vi "Shock&Dyanamics Laboratory - DROPBEAR_June2022_Rev3.vi"() -> ()   [LabVIEW 2019] (continued)
                      tunnel: [T42."Disabled and Grayed Out" ("Disabled") T42."Enabled" ("Disabled")] -> _
                      frame False {
                      }
                      frame True {
                      }
                    }
                  }
                  frame "Voltage", Default {
                  }
                }
                n1114 = case shown="\"Strain\"" w1352 {
                  tunnel: [T42."Enabled" ("Disabled") T42."Disabled and Grayed Out" ("Disabled")] -> w1336
                  frame "Strain" {
                    n1115 = property on="SG Pair 17" class="Bool (strict)"() -> ("Value"=w1457:bool)  [unwired: 2 in, 2 out]
                    n1116 = case shown="True" w1457 {
                      tunnel: [T42."Disabled and Grayed Out" ("Disabled") T42."Enabled" ("Disabled")] -> _
                      frame False {
                      }
                      frame True {
                      }
                    }
                  }
                  frame "Voltage", Default {
                  }
                }
                n1117 = case shown="\"Strain\"" w1350 {
                  tunnel: [T42."Enabled" ("Disabled") T42."Disabled and Grayed Out" ("Disabled")] -> w1334
                  frame "Strain" {
                    n1118 = property on="SG Pair 19" class="Bool (strict)"() -> ("Value"=w1447:bool)  [unwired: 2 in, 2 out]
                    n1119 = case shown="True" w1447 {
                      tunnel: [T42."Disabled and Grayed Out" ("Disabled") T42."Enabled" ("Disabled")] -> _
                      frame False {
                      }
                      frame True {
                      }
                    }
                  }
                  frame "Voltage", Default {
                  }
                }
                n1120 = case shown="\"Strain\"" w1384 {
                  tunnel: [T42."Enabled" ("Disabled") T42."Disabled and Grayed Out" ("Disabled")] -> w1381
                  frame "Strain" {
                    n1121 = property on="SG Pair 1" class="Bool (strict)"() -> ("Value"=w1537:bool)  [unwired: 2 in, 2 out]
                    n1122 = case shown="True" w1537 {
                      tunnel: [T42."Disabled and Grayed Out" ("Disabled") T42."Enabled" ("Disabled")] -> _
                      frame False {
                      }
                      frame True {
                      }
                    }
                  }
                  frame "Voltage", Default {
                  }
                }
                n1123 = case shown="\"Strain\"" w1353 {
                  tunnel: [T42."Enabled" ("Disabled") T42."Disabled and Grayed Out" ("Disabled")] -> w1337
                  frame "Strain" {
                    n1124 = property on="SG Pair 16" class="Bool (strict)"() -> ("Value"=w1462:bool)  [unwired: 2 in, 2 out]
                    n1125 = case shown="True" w1462 {
                      tunnel: [T42."Disabled and Grayed Out" ("Disabled") T42."Enabled" ("Disabled")] -> _
                      frame False {
                      }
                      frame True {
                      }
                    }
                  }
                  frame "Voltage", Default {
                  }
                }
                n1126 = case shown="\"Strain\"" w1355 {
                  tunnel: [T42."Enabled" ("Disabled") T42."Disabled and Grayed Out" ("Disabled")] -> w1360
                  frame "Strain" {
                    n1127 = property on="SG Pair 15" class="Bool (strict)"() -> ("Value"=w1467:bool)  [unwired: 2 in, 2 out]
                    n1128 = case shown="True" w1467 {
                      tunnel: [T42."Disabled and Grayed Out" ("Disabled") T42."Enabled" ("Disabled")] -> _
                      frame False {
                      }
                      frame True {
                      }
                    }
                  }
                  frame "Voltage", Default {
                  }
                }
                n1129 = case shown="\"Strain\"" w1386 {
                  tunnel: [T42."Enabled" ("Disabled") T42."Disabled and Grayed Out" ("Disabled")] -> w1385
                  frame "Strain" {
                    n1130 = property on="SG Pair 0" class="Bool (strict)"() -> ("Value"=w1542:bool)  [unwired: 2 in, 2 out]
                    n1131 = case shown="True" w1542 {
                      tunnel: [T42."Disabled and Grayed Out" ("Disabled") T42."Enabled" ("Disabled")] -> _
                      frame False {
                      }
                      frame True {
                      }
                    }
                  }
                  frame "Voltage", Default {
                  }
                }
                n1132 = case shown="\"Strain\"" w1383 {
                  tunnel: [T42."Enabled" ("Disabled") T42."Disabled and Grayed Out" ("Disabled")] -> w1382
                  frame "Strain" {
                    n1133 = property on="SG Pair 2" class="Bool (strict)"() -> ("Value"=w1532:bool)  [unwired: 2 in, 2 out]
                    n1134 = case shown="True" w1532 {
                      tunnel: [T42."Disabled and Grayed Out" ("Disabled") T42."Enabled" ("Disabled")] -> _
                      frame False {
                      }
                      frame True {
                      }
                    }
                  }
                  frame "Voltage", Default {
                  }
                }
                n1135 = case shown="\"Strain\"" w1376 {
                  tunnel: [T42."Enabled" ("Disabled") T42."Disabled and Grayed Out" ("Disabled")] -> w1373
                  frame "Strain" {
                    n1136 = property on="SG Pair 6" class="Bool (strict)"() -> ("Value"=w1512:bool)  [unwired: 2 in, 2 out]
                    n1137 = case shown="True" w1512 {
                      tunnel: [T42."Disabled and Grayed Out" ("Disabled") T42."Enabled" ("Disabled")] -> _
                      frame False {
                      }
                      frame True {
                      }
                    }
                  }
                  frame "Voltage", Default {
                  }
                }
                n1138 = property on="SG Pair 15" class="Bool (strict)"("DisabledEnum"=w1360) -> ()  [unwired: 2 in, 2 out]
                n1139 = property on="SG Pair 27" class="Bool (strict)"("DisabledEnum"=w1326) -> ()  [unwired: 2 in, 2 out]
                n1140 = property on="SG Pair 17" class="Bool (strict)"("DisabledEnum"=w1336) -> ()  [unwired: 2 in, 2 out]
                n1141 = property on="SG Pair 26" class="Bool (strict)"("DisabledEnum"=w1327) -> ()  [unwired: 2 in, 2 out]
                n1142 = property on="SG Pair 28" class="Bool (strict)"("DisabledEnum"=w1322) -> ()  [unwired: 2 in, 2 out]
                n1143 = property on="SG Pair 23" class="Bool (strict)"("DisabledEnum"=w1330) -> ()  [unwired: 2 in, 2 out]
                n1144 = property on="SG Pair 22" class="Bool (strict)"("DisabledEnum"=w1331) -> ()  [unwired: 2 in, 2 out]
                n1145 = property on="SG Pair 25" class="Bool (strict)"("DisabledEnum"=w1328) -> ()  [unwired: 2 in, 2 out]
                n1146 = property on="SG Pair 16" class="Bool (strict)"("DisabledEnum"=w1337) -> ()  [unwired: 2 in, 2 out]
                n1147 = property on="SG Pair 29" class="Bool (strict)"("DisabledEnum"=w1323) -> ()  [unwired: 2 in, 2 out]
                n1148 = property on="SG Pair 24" class="Bool (strict)"("DisabledEnum"=w1329) -> ()  [unwired: 2 in, 2 out]
                n1149 = property on="SG Pair 19" class="Bool (strict)"("DisabledEnum"=w1334) -> ()  [unwired: 2 in, 2 out]
                n1150 = property on="SG Pair 20" class="Bool (strict)"("DisabledEnum"=w1333) -> ()  [unwired: 2 in, 2 out]
                n1151 = property on="SG Pair 30" class="Bool (strict)"("DisabledEnum"=w1324) -> ()  [unwired: 2 in, 2 out]
                n1152 = property on="SG Pair 31" class="Bool (strict)"("DisabledEnum"=w1325) -> ()  [unwired: 2 in, 2 out]
                n1153 = property on="SG Pair 18" class="Bool (strict)"("DisabledEnum"=w1335) -> ()  [unwired: 2 in, 2 out]
                n1154 = property on="SG Pair 21" class="Bool (strict)"("DisabledEnum"=w1332) -> ()  [unwired: 2 in, 2 out]
                n1155 = property on="SG Pair 0" class="Bool (strict)"("DisabledEnum"=w1385) -> ()  [unwired: 2 in, 2 out]
                n1156 = property on="SG Pair 1" class="Bool (strict)"("DisabledEnum"=w1381) -> ()  [unwired: 2 in, 2 out]
                n1157 = property on="SG Pair 2" class="Bool (strict)"("DisabledEnum"=w1382) -> ()  [unwired: 2 in, 2 out]
                n1158 = property on="SG Pair 3" class="Bool (strict)"("DisabledEnum"=w1379) -> ()  [unwired: 2 in, 2 out]
                n1159 = property on="SG Pair 5" class="Bool (strict)"("DisabledEnum"=w1372) -> ()  [unwired: 2 in, 2 out]
                n1160 = property on="SG Pair 4" class="Bool (strict)"("DisabledEnum"=w1371) -> ()  [unwired: 2 in, 2 out]
                n1161 = property on="SG Pair 9" class="Bool (strict)"("DisabledEnum"=w1369) -> ()  [unwired: 2 in, 2 out]
                n1162 = property on="SG Pair 8" class="Bool (strict)"("DisabledEnum"=w1370) -> ()  [unwired: 2 in, 2 out]
                n1163 = property on="SG Pair 6" class="Bool (strict)"("DisabledEnum"=w1373) -> ()  [unwired: 2 in, 2 out]
                n1164 = property on="SG Pair 7" class="Bool (strict)"("DisabledEnum"=w1374) -> ()  [unwired: 2 in, 2 out]
                n1165 = property on="SG Pair 12" class="Bool (strict)"("DisabledEnum"=w1363) -> ()  [unwired: 2 in, 2 out]
                n1166 = property on="SG Pair 10" class="Bool (strict)"("DisabledEnum"=w1368) -> ()  [unwired: 2 in, 2 out]
                n1167 = property on="SG Pair 11" class="Bool (strict)"("DisabledEnum"=w1364) -> ()  [unwired: 2 in, 2 out]
                n1168 = property on="SG Pair 13" class="Bool (strict)"("DisabledEnum"=w1362) -> ()  [unwired: 2 in, 2 out]
                n1169 = property on="SG Pair 14" class="Bool (strict)"("DisabledEnum"=w1361) -> ()  [unwired: 2 in, 2 out]
              }
              event "Load CH Data": Value Change {
                # "Prompt User to Load CH Data File"
                n1170 = event-data() -> ()  [unwired: 1 in, 5 out]
                n1171 = property on="Folder Name to Save Raw Data" class="Str"() -> ("Value"=w1549:string)  [unwired: 2 in, 2 out]
                n1172 = String To Path(string=w1549) -> (path=w1548:path)
                n1173 = File Dialog(4:"XML File" ("pattern label"), 6:"*.xml" ("pattern"), 7:"Load Channel Data File" ("prompt"), 9:"*.xml" ("default name"), 11:w1548) -> (1:w1551:bool, 3:w1550:path)  [unwired: 2 in, 2 out]
                n1174 = case shown="False" w1551 {
                  tunnel: w1550 -> [w2001 _]
                  frame False {
                    n1175 = call "32CHDAQ - Load Channel Data File.vi"("Channel Data File Path"=w2001) -> ("value"=w1820:T43)  [unwired: 13 in, 1 out]
                    n1176 = Unbundle(w1820) -> ("Value"=w1819:T5)  [unwired: 1 out]
                    n1177 = Unbundle(w1820) -> ("Value"=w2000:T44)  [unwired: 1 out]
                    n1178 = Unbundle(w1819) -> ("Value"=w1818:dbl, "Value"=w1817:dbl)  [unwired: 1 out]
                    n1179 = property on="Striker Velocity (m/s)" class="DigNum (strict)"("Value"=w1818) -> ()  [unwired: 2 in, 2 out]
                    n1180 = property on="Sample Rate (Sa/sec)" class="DigNum (strict)"("Value"=w1817) -> ()  [unwired: 2 in, 2 out]
                    n1181 = Unbundle(w2000) -> (w2052:T45, w2051:T46, w1999:T47, w1998:T48, w1997:T49, w1821:T50, w1996:T51, w1995:T4, w1994:T52, w1652:T53, w1653:T54, w1654:T55)
                    n1182 = Unbundle(w1654) -> ("PF Info"=w1835:string, "PF Info"=w1836:string, "PF Info"=w1837:string, "PF Info"=w1838:string, "PF Info"=w1839:string, "PF Info"=w1840:string, "PF Info"=w1841:string, "PF Info"=w1842:string, "PF Info"=w1843:string, "PF Info"=w1844:string, "PF Info"=w1845:string, "PF Info"=w1846:string, "PF Info"=w1847:string, "PF Info"=w1848:string, "PF Info"=w1849:string, "PF Info"=w1850:string, "PF Info 2"=w1602:string, "PF Info 3"=w1601:string, "PF Info 4"=w1600:string, "PF Info 5"=w1599:string, "PF Info 6"=w1598:string, "PF Info 7"=w1597:string, "PF Info 8"=w1596:string, "PF Info 9"=w1595:string, "PF Info 10"=w1594:string, "PF Info 11"=w1593:string, "PF Info 12"=w1592:string, "PF Info 13"=w1591:string, "PF Info 14"=w1590:string, "PF Info 15"=w1589:string, "PF Info 16"=w1588:string, "PF Info 17"=w1603:string)
                    n1183 = call "32CHDAQ - PF Info Str2Num.vi"("PF Info"=w1835) -> ("PF Channel"=w2047:dbl, "PF Card"=w2048:dbl, "PF Chassis"=w2049:dbl)  [unwired: 2 in]
                    n1184 = call "32CHDAQ - PF Info Str2Num.vi"("PF Info"=w1836) -> ("PF Channel"=w2044:dbl, "PF Card"=w2045:dbl, "PF Chassis"=w2046:dbl)  [unwired: 2 in]
                    n1185 = call "32CHDAQ - PF Info Str2Num.vi"("PF Info"=w1837) -> ("PF Channel"=w2004:dbl, "PF Card"=w2003:dbl, "PF Chassis"=w2002:dbl)  [unwired: 2 in]
                    n1186 = call "32CHDAQ - PF Info Str2Num.vi"("PF Info"=w1838) -> ("PF Channel"=w2007:dbl, "PF Card"=w2006:dbl, "PF Chassis"=w2005:dbl)  [unwired: 2 in]
                    n1187 = call "32CHDAQ - PF Info Str2Num.vi"("PF Info"=w1839) -> ("PF Channel"=w2010:dbl, "PF Card"=w2009:dbl, "PF Chassis"=w2008:dbl)  [unwired: 2 in]
                    n1188 = call "32CHDAQ - PF Info Str2Num.vi"("PF Info"=w1841) -> ("PF Channel"=w2016:dbl, "PF Card"=w2015:dbl, "PF Chassis"=w2014:dbl)  [unwired: 2 in]
                    n1189 = call "32CHDAQ - PF Info Str2Num.vi"("PF Info"=w1842) -> ("PF Channel"=w2019:dbl, "PF Card"=w2018:dbl, "PF Chassis"=w2017:dbl)  [unwired: 2 in]
                    n1190 = call "32CHDAQ - PF Info Str2Num.vi"("PF Info"=w1843) -> ("PF Channel"=w2022:dbl, "PF Card"=w2021:dbl, "PF Chassis"=w2020:dbl)  [unwired: 2 in]
                    n1191 = call "32CHDAQ - PF Info Str2Num.vi"("PF Info"=w1844) -> ("PF Channel"=w2025:dbl, "PF Card"=w2024:dbl, "PF Chassis"=w2023:dbl)  [unwired: 2 in]
                    n1192 = call "32CHDAQ - PF Info Str2Num.vi"("PF Info"=w1845) -> ("PF Channel"=w2028:dbl, "PF Card"=w2027:dbl, "PF Chassis"=w2026:dbl)  [unwired: 2 in]
                    n1193 = call "32CHDAQ - PF Info Str2Num.vi"("PF Info"=w1846) -> ("PF Channel"=w2031:dbl, "PF Card"=w2030:dbl, "PF Chassis"=w2029:dbl)  [unwired: 2 in]
                    n1194 = call "32CHDAQ - PF Info Str2Num.vi"("PF Info"=w1847) -> ("PF Channel"=w2034:dbl, "PF Card"=w2033:dbl, "PF Chassis"=w2032:dbl)  [unwired: 2 in]
                    n1195 = call "32CHDAQ - PF Info Str2Num.vi"("PF Info"=w1848) -> ("PF Channel"=w2037:dbl, "PF Card"=w2036:dbl, "PF Chassis"=w2035:dbl)  [unwired: 2 in]
                    n1196 = call "32CHDAQ - PF Info Str2Num.vi"("PF Info"=w1849) -> ("PF Channel"=w2040:dbl, "PF Card"=w2039:dbl, "PF Chassis"=w2038:dbl)  [unwired: 2 in]
                    n1197 = call "32CHDAQ - PF Info Str2Num.vi"("PF Info"=w1850) -> ("PF Channel"=w2041:dbl, "PF Card"=w2042:dbl, "PF Chassis"=w2043:dbl)  [unwired: 2 in]
                    n1198 = call "32CHDAQ - PF Info Str2Num.vi"("PF Info"=w1602) -> ("PF Channel"=w1649:dbl, "PF Card"=w1650:dbl, "PF Chassis"=w1651:dbl)  [unwired: 2 in]
                    n1199 = call "32CHDAQ - PF Info Str2Num.vi"("PF Info"=w1601) -> ("PF Channel"=w1646:dbl, "PF Card"=w1647:dbl, "PF Chassis"=w1648:dbl)  [unwired: 2 in]
                    n1200 = call "32CHDAQ - PF Info Str2Num.vi"("PF Info"=w1600) -> ("PF Channel"=w1643:dbl, "PF Card"=w1644:dbl, "PF Chassis"=w1645:dbl)  [unwired: 2 in]
                    n1201 = call "32CHDAQ - PF Info Str2Num.vi"("PF Info"=w1599) -> ("PF Channel"=w1640:dbl, "PF Card"=w1641:dbl, "PF Chassis"=w1642:dbl)  [unwired: 2 in]
                    n1202 = call "32CHDAQ - PF Info Str2Num.vi"("PF Info"=w1598) -> ("PF Channel"=w1637:dbl, "PF Card"=w1638:dbl, "PF Chassis"=w1639:dbl)  [unwired: 2 in]
                    n1203 = call "32CHDAQ - PF Info Str2Num.vi"("PF Info"=w1596) -> ("PF Channel"=w1631:dbl, "PF Card"=w1632:dbl, "PF Chassis"=w1633:dbl)  [unwired: 2 in]
                    n1204 = call "32CHDAQ - PF Info Str2Num.vi"("PF Info"=w1595) -> ("PF Channel"=w1628:dbl, "PF Card"=w1629:dbl, "PF Chassis"=w1630:dbl)  [unwired: 2 in]
                    n1205 = call "32CHDAQ - PF Info Str2Num.vi"("PF Info"=w1594) -> ("PF Channel"=w1625:dbl, "PF Card"=w1626:dbl, "PF Chassis"=w1627:dbl)  [unwired: 2 in]
                    n1206 = call "32CHDAQ - PF Info Str2Num.vi"("PF Info"=w1593) -> ("PF Channel"=w1622:dbl, "PF Card"=w1623:dbl, "PF Chassis"=w1624:dbl)  [unwired: 2 in]
                    n1207 = call "32CHDAQ - PF Info Str2Num.vi"("PF Info"=w1592) -> ("PF Channel"=w1619:dbl, "PF Card"=w1620:dbl, "PF Chassis"=w1621:dbl)  [unwired: 2 in]
                    n1208 = call "32CHDAQ - PF Info Str2Num.vi"("PF Info"=w1591) -> ("PF Channel"=w1616:dbl, "PF Card"=w1617:dbl, "PF Chassis"=w1618:dbl)  [unwired: 2 in]
                    n1209 = call "32CHDAQ - PF Info Str2Num.vi"("PF Info"=w1590) -> ("PF Channel"=w1613:dbl, "PF Card"=w1614:dbl, "PF Chassis"=w1615:dbl)  [unwired: 2 in]
                    n1210 = call "32CHDAQ - PF Info Str2Num.vi"("PF Info"=w1589) -> ("PF Channel"=w1610:dbl, "PF Card"=w1611:dbl, "PF Chassis"=w1612:dbl)  [unwired: 2 in]
                    n1211 = call "32CHDAQ - PF Info Str2Num.vi"("PF Info"=w1588) -> ("PF Channel"=w1607:dbl, "PF Card"=w1608:dbl, "PF Chassis"=w1609:dbl)  [unwired: 2 in]
                    n1212 = call "32CHDAQ - PF Info Str2Num.vi"("PF Info"=w1603) -> ("PF Channel"=w1604:dbl, "PF Card"=w1605:dbl, "PF Chassis"=w1606:dbl)  [unwired: 2 in]
                    n1213 = call "32CHDAQ - PF Info Str2Num.vi"("PF Info"=w1840) -> ("PF Channel"=w2013:dbl, "PF Card"=w2012:dbl, "PF Chassis"=w2011:dbl)  [unwired: 2 in]
                    n1214 = call "32CHDAQ - PF Info Str2Num.vi"("PF Info"=w1597) -> ("PF Channel"=w1634:dbl, "PF Card"=w1635:dbl, "PF Chassis"=w1636:dbl)  [unwired: 2 in]
                    n1215 = local write "PF Chassis 26"(w1621) -> ()
                    n1216 = local write "PF Channel 26"(w1619) -> ()
                    n1217 = local write "PF Channel 22"(w1631) -> ()
                    n1218 = local write "PF Chassis 21"(w1636) -> ()
                    n1219 = local write "PF Chassis 27"(w1618) -> ()
                    n1220 = local write "PF Chassis 23"(w1630) -> ()
                    n1221 = local write "PF Channel 23"(w1628) -> ()
                    n1222 = local write "PF Chassis 24"(w1627) -> ()
                    n1223 = local write "PF Channel 24"(w1625) -> ()
                    n1224 = local write "PF Channel 19"(w1640) -> ()
                    n1225 = local write "PF Chassis 20"(w1639) -> ()
                    n1226 = local write "PF Channel 20"(w1637) -> ()
                    n1227 = local write "PF Chassis 22"(w1633) -> ()
                    n1228 = local write "PF Channel 21"(w1634) -> ()
                    n1229 = local write "PF Channel 25"(w1622) -> ()
                    n1230 = local write "PF Channel 18"(w1643) -> ()
                    n1231 = local write "PF Chassis 25"(w1624) -> ()
                    n1232 = local write "PF Card 26"(w1620) -> ()
                    n1233 = local write "PF Chassis 19"(w1642) -> ()
                    n1234 = local write "PF Channel 27"(w1616) -> ()
                    n1235 = local write "PF Channel 28"(w1613) -> ()
                    n1236 = local write "PF Chassis 0"(w2049) -> ()
                    n1237 = local write "PF Card 0"(w2048) -> ()
                    n1238 = local write "PF Channel 0"(w2047) -> ()
                    n1239 = local write "PF Chassis 1"(w2046) -> ()
                    n1240 = local write "PF Card 1"(w2045) -> ()
                    n1241 = local write "PF Channel 1"(w2044) -> ()
                    n1242 = local write "PF Chassis 2"(w2002) -> ()
                    n1243 = local write "PF Card 2"(w2003) -> ()
                    n1244 = local write "PF Channel 2"(w2004) -> ()
                    n1245 = local write "PF Chassis 3"(w2005) -> ()
                    n1246 = local write "PF Card 3"(w2006) -> ()
                    n1247 = local write "PF Channel 3"(w2007) -> ()
                    n1248 = local write "PF Chassis 4"(w2008) -> ()
                    n1249 = local write "PF Card 4"(w2009) -> ()
                    n1250 = local write "PF Channel 4"(w2010) -> ()
                    n1251 = local write "PF Chassis 6"(w2014) -> ()
                    n1252 = local write "PF Card 6"(w2015) -> ()
                    n1253 = local write "PF Channel 6"(w2016) -> ()
                    n1254 = local write "PF Chassis 7"(w2017) -> ()
                    n1255 = local write "PF Card 7"(w2018) -> ()
                    n1256 = local write "PF Channel 7"(w2019) -> ()
                    n1257 = local write "PF Chassis 8"(w2020) -> ()
                    n1258 = local write "PF Channel 8"(w2021) -> ()
                    n1259 = local write "PF Card 8"(w2022) -> ()
                    n1260 = local write "PF Chassis 9"(w2023) -> ()
                    n1261 = local write "PF Card 9"(w2024) -> ()
                    n1262 = local write "PF Channel 9"(w2025) -> ()
                    n1263 = local write "PF Chassis 10"(w2026) -> ()
                    n1264 = local write "PF Card 10"(w2027) -> ()
                    n1265 = local write "PF Channel 10"(w2028) -> ()
                    n1266 = local write "PF Chassis 11"(w2029) -> ()
                    n1267 = local write "PF Card 11"(w2030) -> ()
                    n1268 = local write "PF Channel 11"(w2031) -> ()
                    n1269 = local write "PF Chassis 12"(w2032) -> ()
                    n1270 = local write "PF Card 12"(w2033) -> ()
                    n1271 = local write "PF Channel 12"(w2034) -> ()
                    n1272 = local write "PF Chassis 13"(w2035) -> ()
                    n1273 = local write "PF Card 13"(w2036) -> ()
                    n1274 = local write "PF Channel 13"(w2037) -> ()
                    n1275 = local write "PF Chassis 14"(w2038) -> ()
                    n1276 = local write "PF Card 14"(w2039) -> ()
                    n1277 = local write "PF Channel 14"(w2040) -> ()
                    n1278 = local write "PF Chassis 15"(w2043) -> ()
                    n1279 = local write "PF Card 15"(w2042) -> ()
                    n1280 = local write "PF Channel 15"(w2041) -> ()
                    n1281 = local write "PF Channel 17"(w1646) -> ()
                    n1282 = local write "PF Chassis 28"(w1615) -> ()
                    n1283 = local write "PF Chassis 29"(w1612) -> ()
                    n1284 = local write "PF Chassis 16"(w1651) -> ()
                    n1285 = local write "PF Channel 16"(w1649) -> ()
                    n1286 = local write "PF Chassis 18"(w1645) -> ()
                    n1287 = local write "PF Channel 29"(w1610) -> ()
                    n1288 = local write "PF Chassis 30"(w1609) -> ()
                    n1289 = local write "PF Chassis 17"(w1648) -> ()
                    n1290 = local write "PF Card 23"(w1629) -> ()
                    n1291 = local write "PF Channel 30"(w1607) -> ()
                    n1292 = local write "PF Card 21"(w1635) -> ()
                    n1293 = local write "PF Card 24"(w1626) -> ()
                    n1294 = local write "PF Chassis 5"(w2011) -> ()
                    n1295 = local write "PF Card 5"(w2012) -> ()
                    n1296 = local write "PF Channel 5"(w2013) -> ()
                    n1297 = local write "PF Card 22"(w1632) -> ()
                    n1298 = local write "PF Card 16"(w1650) -> ()
                    n1299 = local write "PF Card 20"(w1638) -> ()
                    n1300 = local write "PF Card 27"(w1617) -> ()
                    n1301 = local write "PF Chassis 31"(w1606) -> ()
                    n1302 = local write "PF Card 17"(w1647) -> ()
                    n1303 = local write "PF Card 19"(w1641) -> ()
                    n1304 = local write "PF Card 28"(w1614) -> ()
                    n1305 = local write "PF Card 29"(w1611) -> ()
                    n1306 = local write "PF Card 18"(w1644) -> ()
                    n1307 = local write "PF Card 25"(w1623) -> ()
                    n1308 = local write "PF Card 30"(w1608) -> ()
                    n1309 = local write "PF Channel 31"(w1604) -> ()
                    n1310 = Unbundle(w2052) -> ("Enable Ch 1"=w1834:bool, "Enable Ch 2"=w1833:bool, "Enable Ch 3"=w1832:bool, "Enable Ch 4"=w1831:bool, "Enable Ch 5"=w1830:bool, "Enable Ch 6"=w1829:bool, "Enable Ch 7"=w1828:bool, "Enable Ch 8"=w1827:bool, "Enable Ch 9"=w1826:bool, "Enable Ch 10"=w1825:bool, "Enable Ch 11"=w1824:bool, "Enable Ch 12"=w1823:bool, "Enable Ch 13"=w1822:bool, "Enable Ch 14"=w1816:bool, "Enable Ch 15"=w1815:bool, "Enable Ch 16"=w1814:bool, "Enable Ch 17"=w1813:bool, "Enable Ch 18"=w1812:bool, "Enable Ch 19"=w1811:bool, "Enable Ch 20"=w1810:bool, "Enable Ch 21"=w1799:bool, "Enable Ch 22"=w1800:bool, "Enable Ch 23"=w1801:bool, "Enable Ch 24"=w1802:bool, "Enable Ch 25"=w1803:bool, "Enable Ch 26"=w1804:bool, "Enable Ch 27"=w1805:bool, "Enable Ch 28"=w1806:bool, "Enable Ch 29"=w1807:bool, "Enable Ch 30"=w1808:bool, w1809:bool)  [unwired: 1 out]
                    n1311 = local write "PF Card 31"(w1605) -> ()
                    n1312 = property on="Enable Ch 12" class="Bool (strict)"("Value"=w1823) -> ()  [unwired: 2 in, 2 out]
                    n1313 = property on="Enable Ch 13" class="Bool (strict)"("Value"=w1822) -> ()  [unwired: 2 in, 2 out]
                    n1314 = property on="Enable Ch 15" class="Bool (strict)"("Value"=w1815) -> ()  [unwired: 2 in, 2 out]
                    n1315 = property on="Enable Ch 11" class="Bool (strict)"("Value"=w1824) -> ()  [unwired: 2 in, 2 out]
                    n1316 = property on="Enable Ch 14" class="Bool (strict)"("Value"=w1816) -> ()  [unwired: 2 in, 2 out]
                    n1317 = property on="Enable Ch 10" class="Bool (strict)"("Value"=w1825) -> ()  [unwired: 2 in, 2 out]
                    n1318 = property on="Enable Ch 9" class="Bool (strict)"("Value"=w1826) -> ()  [unwired: 2 in, 2 out]
                    n1319 = property on="Enable Ch 6" class="Bool (strict)"("Value"=w1829) -> ()  [unwired: 2 in, 2 out]
                    n1320 = property on="Enable Ch 4" class="Bool (strict)"("Value"=w1831) -> ()  [unwired: 2 in, 2 out]
                    n1321 = property on="Enable Ch 5" class="Bool (strict)"("Value"=w1830) -> ()  [unwired: 2 in, 2 out]
                    n1322 = property on="Enable Ch 7" class="Bool (strict)"("Value"=w1828) -> ()  [unwired: 2 in, 2 out]
                    n1323 = property on="Enable Ch 8" class="Bool (strict)"("Value"=w1827) -> ()  [unwired: 2 in, 2 out]
                    n1324 = property on="Enable Ch 3" class="Bool (strict)"("Value"=w1832) -> ()  [unwired: 2 in, 2 out]
                    n1325 = property on="Enable Ch 1" class="Bool (strict)"("Value"=w1834) -> ()  [unwired: 2 in, 2 out]
                    n1326 = property on="Enable Ch 2" class="Bool (strict)"("Value"=w1833) -> ()  [unwired: 2 in, 2 out]
                    n1327 = local write "LED Enable Ch 18"(w1812) -> ()
                    n1328 = local write "LED Enable Ch 16"(w1814) -> ()
                    n1329 = local write "LED Enable Ch 12"(w1823) -> ()
                    n1330 = local write "LED Enable Ch 17"(w1813) -> ()
                    n1331 = local write "LED Enable Ch 19"(w1811) -> ()
                    n1332 = local write "LED Enable Ch 9"(w1826) -> ()
                    n1333 = local write "LED Enable Ch 13"(w1822) -> ()
                    n1334 = local write "LED Enable Ch 20"(w1810) -> ()
                    n1335 = local write "LED Enable Ch 10"(w1825) -> ()
                    n1336 = local write "LED Enable Ch 11"(w1824) -> ()
                    n1337 = local write "LED Enable Ch 6"(w1829) -> ()
                    n1338 = local write "LED Enable Ch 7"(w1828) -> ()
                    n1339 = local write "LED Enable Ch 5"(w1830) -> ()
                    n1340 = local write "LED Enable Ch 8"(w1827) -> ()
                    n1341 = local write "LED Enable Ch 4"(w1831) -> ()
                    n1342 = local write "LED Enable Ch 3"(w1832) -> ()
                    n1343 = local write "LED Enable Ch 14"(w1816) -> ()
                    n1344 = local write "LED Enable Ch 15"(w1815) -> ()
                    n1345 = local write "LED Enable Ch 1"(w1834) -> ()
                    n1346 = local write "LED Enable Ch 2"(w1833) -> ()
                    n1347 = local write "LED Enable Ch 22"(w1800) -> ()
                    n1348 = local write "LED Enable Ch 23"(w1801) -> ()
                    n1349 = local write "LED Enable Ch 24"(w1802) -> ()
                    n1350 = local write "LED Enable Ch 21"(w1799) -> ()
                    n1351 = Unbundle(w1653) -> ("PF Condition 0"=w1866:bool, "PF Condition 1"=w1863:bool, "PF Condition 2"=w1861:bool, "PF Condition 3"=w1860:bool, "PF Condition 4"=w1859:bool, "PF Condition 5"=w1854:bool, "PF Condition 6"=w1853:bool, "PF Condition 7"=w1852:bool, "PF Condition 8"=w1851:bool, "PF Condition 9"=w1855:bool, "PF Condition 10"=w1856:bool, "PF Condition 11"=w1857:bool, "PF Condition 12"=w1858:bool, "PF Condition 13"=w1862:bool, "PF Condition 14"=w1864:bool, "PF Condition 15"=w1865:bool, "PF Condition 16"=w1686:bool, "PF Condition 17"=w1685:bool, "PF Condition 18"=w1684:bool, "PF Condition 19"=w1683:bool, "PF Condition 20"=w1682:bool, "PF Condition 21"=w1681:bool, "PF Condition 22"=w1680:bool, "PF Condition 23"=w1679:bool, "PF Condition 24"=w1678:bool, "PF Condition 25"=w1677:bool, "PF Condition 26"=w1676:bool, "PF Condition 27"=w1675:bool, "PF Condition 28"=w1674:bool, "PF Condition 29"=w1673:bool, "PF Condition 30"=w1672:bool, "PF Condition 31"=w1671:bool)
                    n1352 = local write "LED Enable Ch 25"(w1803) -> ()
                    n1353 = local write "LED Enable Ch 26"(w1804) -> ()
                    n1354 = local write "LED Enable Ch 28"(w1806) -> ()
                    n1355 = local write "LED Enable Ch 27"(w1805) -> ()
                    n1356 = local write "LED Enable Ch 29"(w1807) -> ()
                    n1357 = local write "LED Enable Ch 30"(w1808) -> ()
                    n1358 = local write "LED Enable Ch 31"(w1809) -> ()
                    n1359 = local write "PF Condition 0"(w1866) -> ()
                    n1360 = local write "PF Condition 1"(w1863) -> ()
                    n1361 = local write "PF Condition 2"(w1861) -> ()
                    n1362 = local write "PF Condition 3"(w1860) -> ()
                    n1363 = local write "PF Condition 4"(w1859) -> ()
                    n1364 = local write "PF Condition 5"(w1854) -> ()
                    n1365 = local write "PF Condition 6"(w1853) -> ()
                    n1366 = local write "PF Condition 7"(w1852) -> ()
                    n1367 = local write "PF Condition 8"(w1851) -> ()
                    n1368 = local write "PF Condition 9"(w1855) -> ()
                    n1369 = local write "PF Condition 10"(w1856) -> ()
                    n1370 = local write "PF Condition 11"(w1857) -> ()
                    n1371 = local write "PF Condition 12"(w1858) -> ()
                    n1372 = local write "PF Condition 13"(w1862) -> ()
                    n1373 = local write "PF Condition 14"(w1864) -> ()
                    n1374 = local write "PF Condition 15"(w1865) -> ()
                    n1375 = local write "PF Condition 28"(w1674) -> ()
                    n1376 = local write "PF Condition 29"(w1673) -> ()
                    n1377 = local write "PF Condition 23"(w1679) -> ()
                    n1378 = local write "PF Condition 16"(w1686) -> ()
                    n1379 = local write "PF Condition 20"(w1682) -> ()
                    n1380 = local write "PF Condition 21"(w1681) -> ()
                    n1381 = local write "PF Condition 24"(w1678) -> ()
                    n1382 = local write "PF Condition 17"(w1685) -> ()
                    n1383 = local write "PF Condition 18"(w1684) -> ()
                    n1384 = local write "PF Condition 22"(w1680) -> ()
                    n1385 = local write "PF Condition 25"(w1677) -> ()
                    n1386 = local write "PF Condition 26"(w1676) -> ()
                    n1387 = local write "PF Condition 27"(w1675) -> ()
                    n1388 = local write "PF Condition 19"(w1683) -> ()
                    n1389 = local write "PF Condition 30"(w1672) -> ()
                    n1390 = local write "PF Condition 31"(w1671) -> ()
                    n1391 = Unbundle(w2051) -> ("Name (Trigger Channel)"=w2050:string, "Name Ch 1"=w1979:string, "Name Ch 2"=w1980:string, "Name Ch 3"=w1981:string, "Name Ch4"=w1982:string, "Name Ch 5"=w1983:string, "Name Ch 6"=w1984:string, "Name Ch 7"=w1985:string, "Name Ch 8"=w1986:string, "Name Ch 9"=w1987:string, "Name Ch 10"=w1988:string, "Name Ch 11"=w1989:string, "Name Ch 12"=w1990:string, "Name Ch 13"=w1991:string, "Name Ch 14"=w1992:string, "Name Ch 15"=w1993:string, "Name Ch 16"=w1798:string, "Name Ch 17"=w1797:string, "Name Ch 18"=w1796:string, "Name Ch 19"=w1795:string, "Name Ch 20"=w1794:string, "Name Ch 21"=w1793:string, "Name Ch 22"=w1792:string, "Name Ch 23"=w1791:string, "Name Ch 24"=w1790:string, "Name Ch 25"=w1789:string, "Name Ch 26"=w1788:string, "Name Ch4 2"=w1787:string, "Name Ch 4"=w1786:string, "Name Ch 27"=w1785:string, "Name Ch 28"=w1784:string, "Name (Trigger Channel) 2"=w1783:string)
                    n1392 = local write "Name Ch 4"(w1982) -> ()
                    n1393 = local write "Name Ch 1"(w1979) -> ()
                    n1394 = local write "Name Ch 2"(w1980) -> ()
                    n1395 = local write "Name Ch 3"(w1981) -> ()
                    n1396 = local write "Name Ch 5"(w1983) -> ()
                    n1397 = local write "Name Ch 6"(w1984) -> ()
                    n1398 = local write "Name Ch 7"(w1985) -> ()
                    n1399 = local write "Name Ch 8"(w1986) -> ()
                    n1400 = local write "Name Ch 9"(w1987) -> ()
                    n1401 = local write "Name Ch 10"(w1988) -> ()
                    n1402 = local write "Name Ch 11"(w1989) -> ()
                    n1403 = local write "Name Ch 12"(w1990) -> ()
                    n1404 = local write "Name Ch 13"(w1991) -> ()
                    n1405 = local write "Name Ch 14"(w1992) -> ()
                    n1406 = local write "Name Ch 15"(w1993) -> ()
                    n1407 = local write "Name (Laser Gate)"(w2050) -> ()
                    n1408 = local write "Name Ch 18"(w1796) -> ()
                    n1409 = local write "Name Ch 19"(w1795) -> ()
                    n1410 = local write "Name Ch 16"(w1798) -> ()
                    n1411 = local write "Name Ch 17"(w1797) -> ()
                    n1412 = local write "Name Ch 21"(w1793) -> ()
                    n1413 = local write "Name Ch 20"(w1794) -> ()
                    n1414 = local write "Name Ch 22"(w1792) -> ()
                    n1415 = local write "Name Ch 23"(w1791) -> ()
                    n1416 = local write "Name Ch 31"(w1783) -> ()
                    n1417 = local write "Name Ch 24"(w1790) -> ()
                    n1418 = local write "Name Ch 26"(w1788) -> ()
                    n1419 = local write "Name Ch 27"(w1787) -> ()
                    n1420 = local write "Name Ch 28"(w1786) -> ()
                    n1421 = local write "Name Ch 25"(w1789) -> ()
                    n1422 = local write "Name Ch 30"(w1784) -> ()
                    n1423 = local write "Name Ch 29"(w1785) -> ()
                    n1424 = Unbundle(w1999) -> ("Physical Channels Ch0"=w1978:tag, "Physical Channel Ch 1"=w1971:tag, "Physical Channel Ch 2"=w1970:tag, "Physical Channels Ch 3"=w1969:tag, "Physical Channel Ch 4"=w1968:tag, "Physical Channel Ch 5"=w1967:tag, "Physical Channels Ch 6"=w1966:tag, "Physical Channel Ch 7"=w1965:tag, "Physical Channel Ch 8"=w1964:tag, "Physical Channel Ch 9"=w1963:tag, "Physical Channel Ch 10"=w1972:tag, "Physical Channel Ch 11"=w1973:tag, "Physical Channel Ch 12"=w1974:tag, "Physical Channel Ch 13"=w1975:tag, "Physical Channel Ch 14"=w1976:tag, "Physical Channel Ch 15"=w1977:tag, "Physical Channel Ch 16"=w1782:tag, "Physical Channel Ch 17"=w1781:tag, "Physical Channel Ch 18"=w1780:tag, "Physical Channel Ch 19"=w1779:tag, "Physical Channel Ch 20"=w1778:tag, "Physical Channel Ch 21"=w1777:tag, "Physical Channel Ch 22"=w1776:tag, "Physical Channel Ch 23"=w1775:tag, "Physical Channel Ch 24"=w1774:tag, "Physical Channels Ch 7"=w1773:tag, "Physical Channel Ch 6"=w1772:tag, "Physical Channel Ch 25"=w1771:tag, "Physical Channels Ch 4"=w1770:tag, "Physical Channel Ch 3"=w1769:tag, "Physical Channel Ch 26"=w1768:tag, "Physical Channels Ch0 2"=w1767:tag)
                    n1425 = local write "Physical Channel Ch 16"(w1782) -> ()
                    n1426 = local write "Physical Channel Ch 18"(w1780) -> ()
                    n1427 = local write "Physical Channel Ch 19"(w1779) -> ()
                    n1428 = local write "Physical Channel Ch 21"(w1777) -> ()
                    n1429 = local write "Physical Channel Ch 20"(w1778) -> ()
                    n1430 = local write "Physical Channel Ch 24"(w1774) -> ()
                    n1431 = local write "Physical Channel Ch 17"(w1781) -> ()
                    n1432 = local write "Physical Channel Ch 22"(w1776) -> ()
                    n1433 = local write "Physical Channel Ch 23"(w1775) -> ()
                    n1434 = local write "Physical Channel Ch 26"(w1772) -> ()
                    n1435 = local write "Physical Channel Ch 25"(w1773) -> ()
                    n1436 = local write "Physical Channel Ch 29"(w1769) -> ()
                    n1437 = local write "Physical Channel Ch 28"(w1770) -> ()
                    n1438 = local write "Physical Channel Ch 30"(w1768) -> ()
                    n1439 = local write "Physical Channel Ch 27"(w1771) -> ()
                    n1440 = local write "Physical Channel Ch 31"(w1767) -> ()
                    n1441 = Unbundle(w1652) -> ("SG Pair Ch 0"=w1587:T9, "SG Pair Ch 1"=w1586:T10, "SG Pair Ch 2"=w1585:T11, "SG Pair Ch 3"=w1584:T12, "SG Pair Ch 4"=w1583:T13, "SG Pair Ch 5"=w1582:T14, "SG Pair Ch 6"=w1581:T15, "SG Pair Ch 7"=w1580:T16, "SG Pair Ch 8"=w1579:T17, "SG Pair Ch 9"=w1578:T18, "SG Pair Ch 10"=w1577:T19, "SG Pair Ch 11"=w1576:T20, "SG Pair Ch 12"=w1575:T21, "SG Pair Ch 13"=w1574:T22, "SG Pair Ch 14"=w1573:T23, "SG Pair Ch 15"=w1572:T24, "SG Pair Ch 16"=w1571:T25, "SG Pair Ch 17"=w1570:T26, "SG Pair Ch 18"=w1569:T27, "SG Pair Ch 19"=w1568:T28, "SG Pair Ch 20"=w1567:T29, "SG Pair Ch 21"=w1566:T30, "SG Pair Ch 22"=w1565:T31, "SG Pair Ch 23"=w1564:T32, "SG Pair Ch 24"=w1563:T33, "SG Pair Ch 25"=w1562:T34, "SG Pair Ch 26"=w1561:T35, "SG Pair Ch 27"=w1560:T36, "SG Pair Ch 28"=w1559:T37, "SG Pair Ch 29"=w1558:T38, "SG Pair Ch 30"=w1557:T39, "SG Pair Ch 31"=w1556:T40)
                    n1442 = local write "Physical Channels Ch 0"(w1978) -> ()
                    n1443 = local write "Physical Channel Ch 1"(w1971) -> ()
                    n1444 = local write "Physical Channel Ch 2"(w1970) -> ()
                    n1445 = local write "Physical Channels Ch 3"(w1969) -> ()
                    n1446 = local write "Physical Channel Ch 4"(w1968) -> ()
                    n1447 = local write "Physical Channel Ch 5"(w1967) -> ()
                    n1448 = local write "Physical Channels Ch 6"(w1966) -> ()
                    n1449 = local write "Physical Channel Ch 7"(w1965) -> ()
                    n1450 = local write "Physical Channel Ch 8"(w1964) -> ()
                    n1451 = local write "Physical Channel Ch 9"(w1963) -> ()
                    n1452 = local write "Physical Channel Ch 10"(w1972) -> ()
                    n1453 = local write "Physical Channel Ch 11"(w1973) -> ()
                    n1454 = local write "Physical Channel Ch 12"(w1974) -> ()
                    n1455 = local write "Physical Channel Ch 13"(w1975) -> ()
                    n1456 = local write "Physical Channel Ch 14"(w1976) -> ()
                    n1457 = local write "Physical Channel Ch 15"(w1977) -> ()
                    n1458 = local write "SG Pair Ch 2"(w1585) -> ()
                    n1459 = local write "SG Pair Ch 3"(w1584) -> ()
                    n1460 = local write "SG Pair Ch 1"(w1586) -> ()
                    n1461 = local write "SG Pair Ch 6"(w1581) -> ()
                    n1462 = local write "SG Pair Ch 4"(w1583) -> ()
                    n1463 = local write "SG Pair Ch 10"(w1577) -> ()
                    n1464 = local write "SG Pair Ch 5"(w1582) -> ()
                    n1465 = local write "SG Pair Ch 7"(w1580) -> ()
                    n1466 = local write "SG Pair Ch 8"(w1579) -> ()
                    n1467 = local write "SG Pair Ch 14"(w1573) -> ()
                    n1468 = local write "SG Pair Ch 11"(w1576) -> ()
                    n1469 = local write "SG Pair Ch 12"(w1575) -> ()
                    n1470 = local write "SG Pair Ch 0"(w1587) -> ()
                    n1471 = local write "SG Pair Ch 9"(w1578) -> ()
                    n1472 = local write "SG Pair Ch 13"(w1574) -> ()
                    n1473 = local write "SG Pair Ch 15"(w1572) -> ()
                    n1474 = local write "SG Pair Ch 16"(w1571) -> ()
                    n1475 = local write "SG Pair Ch 17"(w1570) -> ()
                    n1476 = local write "SG Pair Ch 18"(w1569) -> ()
                    n1477 = local write "SG Pair Ch 19"(w1568) -> ()
                    n1478 = local write "SG Pair Ch 20"(w1567) -> ()
                    n1479 = local write "SG Pair Ch 21"(w1566) -> ()
                    n1480 = local write "SG Pair Ch 22"(w1565) -> ()
                    n1481 = local write "SG Pair Ch 23"(w1564) -> ()
                    n1482 = local write "SG Pair Ch 24"(w1563) -> ()
                    n1483 = local write "SG Pair Ch 25"(w1562) -> ()
                    n1484 = local write "SG Pair Ch 29"(w1558) -> ()
